vi "testConfigServersAandB.vi"(8 "error in (no error)":errorcluster) -> (0 "error out":errorcluster)   [LabVIEW 2018]
doc: "Test the configServer.vi for TCP/IP servers A and B."
uses:
  src/TcpServer/TcpServer.lvclass
  src/TcpServerTel/typedef/enqueueOptionsTypeDef.ctl
  src/TcpServer/configServerTypeDef.ctl
  src/TcpServer/TcpServer.lvclass/TcpServer.ctl
  src/TcpServerBase/TcpServerBase.lvclass/TcpServerBase.ctl
  src/TcpServerTel/TcpServerTel.lvclass/TcpServerTel.ctl
  src/TcpServerCmd/TcpServerCmd.lvclass
  home/pcortes/Documents/github/ts_labview_tcp_json/src/TcpServerBase/TcpServerBase.lvclass
  src/TcpServerTel/TcpServerTel.lvclass
  <vilib>/addons/_JKI Toolkits/Caraya/classes/Assert/Assert Not Equal Value_Variant.vi
  <vilib>/addons/_JKI Toolkits/Caraya/classes/Assert/Assert Equal Value_Variant.vi
  <vilib>/addons/_JKI Toolkits/Caraya/classes/Test/Test.lvclass
  <vilib>/addons/_JKI Toolkits/Caraya/classes/Assert/Assert.lvclass
  src/TcpServerBase/TcpServerBase.lvclass
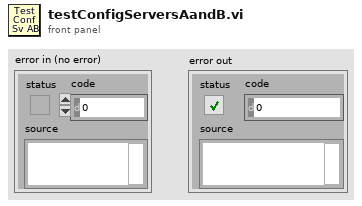
[diagram p1: front panel]
types:
  T1 = typedef "TcpServerTel.lvclass/enqueueOptionsTypeDef.ctl" = enum16{"lossy enqueue", "normal enqueue"}
  T2 = typedef "TcpServer.lvclass/configServerTypeDef.ctl" = cluster{"cmdServerPort":u16, "telServerPort":u16, "timeoutServerInMs":i32, "serverBytesToRead":i32, "maxSizeQueueTcpClientFromDds":i32, "EnqueueOptions":T1, "timeoutQueueTcpClientFromDds (ms)":i32, "maxSizeQueueTcpClient":i32, "timeoutInMs":i32}
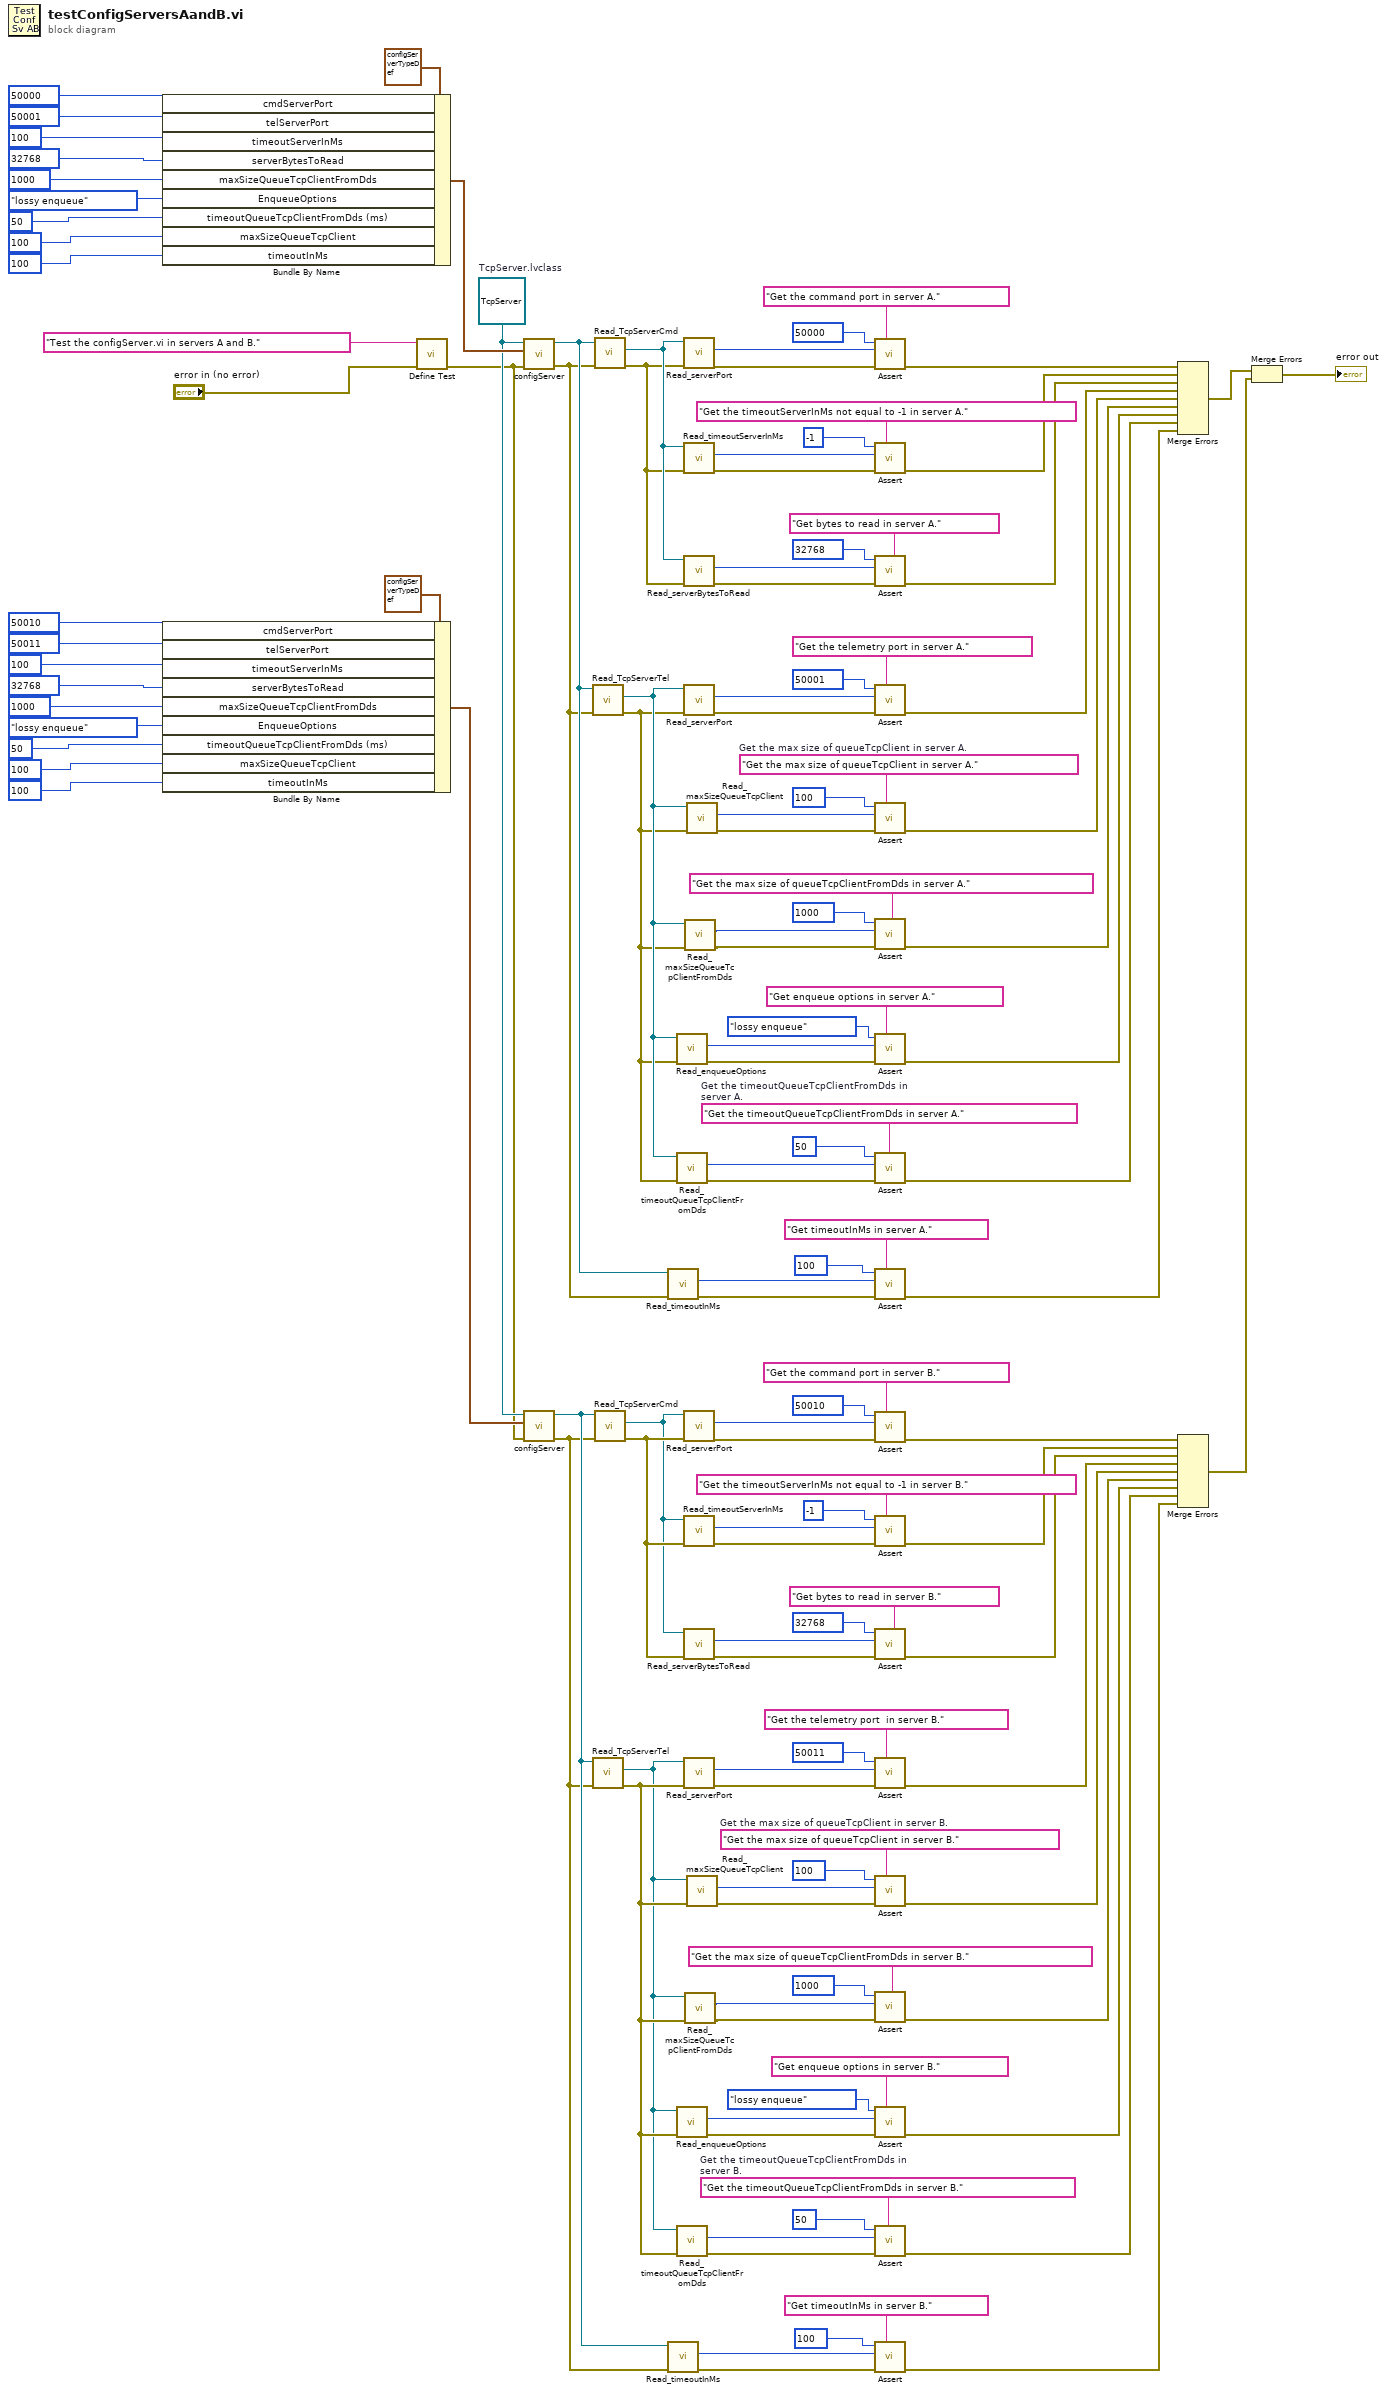
[diagram p0: block diagram]
diagram:
  w34 = "Get the max size of queueTcpClient in server B."  # Get the max size of queueTcpClient in server B.
  w31 = "Get the timeoutQueueTcpClientFromDds in server B."  # Get the timeoutQueueTcpClientFromDds in server B.
  w104 = "Get the max size of queueTcpClient in server A."  # Get the max size of queueTcpClient in server A.
  w107 = "Get the timeoutQueueTcpClientFromDds in server A."  # Get the timeoutQueueTcpClientFromDds in server A.
  w58 = refnum<class "TcpServer.lvclass"> refnum  # TcpServer.lvclass
  n1 = Bundle By Name(cluster=T2 {"cmdServerPort"=8888, "telServerPort"=8889, "timeoutServerInMs"=100, "serverBytesToRead"=32768, "maxSizeQueueTcpClientFromDds"=1000, "EnqueueOptions"=enum."lossy enqueue", "timeoutQueueTcpClientFromDds (ms)"=50, "maxSizeQueueTcpClient"=1000, "timeoutInMs"=100} ("ServerConfiguration"), "cmdServerPort"=u16 50000, "telServerPort"=u16 50001, "timeoutServerInMs"=100 ("serverTimeout (ms)"), "serverBytesToRead"=32768, "maxSizeQueueTcpClientFromDds"=1000 ("telQueueServerMaxSize"), "EnqueueOptions"=enqueueOptionsTypeDef."lossy enqueue", "timeoutQueueTcpClientFromDds (ms)"=50 ("telQueueServerTimeout"), "maxSizeQueueTcpClient"=100 ("tcpClientQueueMaxSize"), "timeoutInMs"=100 ("timeoutStatusNotifier")) -> (w69:T2)
  n2 = Bundle By Name(cluster=T2 {"cmdServerPort"=8888, "telServerPort"=8889, "timeoutServerInMs"=100, "serverBytesToRead"=32768, "maxSizeQueueTcpClientFromDds"=1000, "EnqueueOptions"=enum."lossy enqueue", "timeoutQueueTcpClientFromDds (ms)"=50, "maxSizeQueueTcpClient"=1000, "timeoutInMs"=100} ("ServerConfiguration"), "cmdServerPort"=u16 50010, "telServerPort"=u16 50011, "timeoutServerInMs"=100 ("serverTimeout (ms)"), "serverBytesToRead"=32768, "maxSizeQueueTcpClientFromDds"=1000 ("telQueueServerMaxSize"), "EnqueueOptions"=enqueueOptionsTypeDef."lossy enqueue", "timeoutQueueTcpClientFromDds (ms)"=50 ("telQueueServerTimeout"), "maxSizeQueueTcpClient"=100 ("tcpClientQueueMaxSize"), "timeoutInMs"=100 ("timeoutStatusNotifier")) -> (w8:T2)
  n3 = call <vilib>:"Define Test.vi"("error in (no error)"="error in (no error)", "Label (VI Title)"="Test the configServer.vi in servers A and B.") -> ("error out"=w1:errorcluster)  [unwired: 9 in]
  n4 = call "configServer.vi"("error in (no error)"=w1, "ServerConfiguration"=w69, "tcpServer in"=w58) -> ("error out"=w79:errorcluster, "tcpServer out"=w80:refnum<class "TcpServer.lvclass">)  [unwired: 7 in]
  n5 = call "configServer.vi"("error in (no error)"=w1, "ServerConfiguration"=w8, "tcpServer in"=w58) -> ("error out"=w2:errorcluster, "tcpServer out"=w3:refnum<class "TcpServer.lvclass">)  [unwired: 7 in]
  n6 = call "Read_TcpServerTel.vi"("error in (no error)"=w79, "TcpServer in"=w80) -> ("error out"=w71:errorcluster, "TcpServerTel.lvclass"=w72:refnum<class "TcpServerTel.lvclass">)  [unwired: 7 in, 1 out]
  n7 = call "Read_TcpServerTel.vi"("error in (no error)"=w2, "TcpServer in"=w3) -> ("error out"=w56:errorcluster, "TcpServerTel.lvclass"=w55:refnum<class "TcpServerTel.lvclass">)  [unwired: 7 in, 1 out]
  n8 = call "Read_TcpServerCmd.vi"("error in (no error)"=w79, "TcpServer in"=w80) -> ("error out"=w74:errorcluster, "TcpServerCmd.lvclass"=w75:refnum<class "TcpServerCmd.lvclass">)  [unwired: 7 in, 1 out]
  n9 = call "Read_TcpServerCmd.vi"("error in (no error)"=w2, "TcpServer in"=w3) -> ("error out"=w53:errorcluster, "TcpServerCmd.lvclass"=w52:refnum<class "TcpServerCmd.lvclass">)  [unwired: 7 in, 1 out]
  n10 = call "Read_timeoutInMs.vi"("error in (no error)"=w79, "TcpServer in"=w80) -> ("error out"=w78:errorcluster, "timeoutInMs"=w77:i32)  [unwired: 7 in, 1 out]
  n11 = call "Read_timeoutInMs.vi"("error in (no error)"=w2, "TcpServer in"=w3) -> ("error out"=w49:errorcluster, "timeoutInMs"=w50:i32)  [unwired: 7 in, 1 out]
  n12 = call "Read_enqueueOptions.vi"("error in (no error)"=w71, "TcpServerTel in"=w72) -> ("error out"=w99:errorcluster, "EnqueueOptions"=w98:T1)  [unwired: 7 in, 1 out]
  n13 = call "Read_timeoutQueueTcpClientFromDds.vi"("error in (no error)"=w71, "TcpServerTel in"=w72) -> ("error out"=w97:errorcluster, "timeoutQueueTcpClientFromDds"=w96:i32)  [unwired: 7 in, 1 out]
  n14 = call "Read_enqueueOptions.vi"("error in (no error)"=w56, "TcpServerTel in"=w55) -> ("error out"=w39:errorcluster, "EnqueueOptions"=w40:T1)  [unwired: 7 in, 1 out]
  n15 = call "Read_timeoutQueueTcpClientFromDds.vi"("error in (no error)"=w56, "TcpServerTel in"=w55) -> ("error out"=w41:errorcluster, "timeoutQueueTcpClientFromDds"=w42:i32)  [unwired: 7 in, 1 out]
  n16 = call "Read_serverPort.vi"("error in (no error)"=w74, "TcpServerBase in"=w75) -> ("error out"=w127:errorcluster, "serverPort"=w126:u16)  [unwired: 7 in, 1 out]
  n17 = call "Read_timeoutServerInMs.vi"("error in (no error)"=w74, "TcpServerBase in"=w75) -> ("error out"=w122:errorcluster, "timeoutServerInMs"=w123:i32)  [unwired: 7 in, 1 out]
  n18 = call "Read_serverBytesToRead.vi"("error in (no error)"=w74, "TcpServerBase in"=w75) -> ("error out"=w117:errorcluster, "serverBytesToRead"=w116:i32)  [unwired: 7 in, 1 out]
  n19 = call "Read_serverPort.vi"("error in (no error)"=w71, "TcpServerBase in"=w72) -> ("error out"=w112:errorcluster, "serverPort"=w111:u16)  [unwired: 7 in, 1 out]
  n20 = call "Read_serverPort.vi"("error in (no error)"=w53, "TcpServerBase in"=w52) -> ("error out"=w11:errorcluster, "serverPort"=w12:u16)  [unwired: 7 in, 1 out]
  n21 = call "Read_timeoutServerInMs.vi"("error in (no error)"=w53, "TcpServerBase in"=w52) -> ("error out"=w16:errorcluster, "timeoutServerInMs"=w15:i32)  [unwired: 7 in, 1 out]
  n22 = call "Read_serverBytesToRead.vi"("error in (no error)"=w53, "TcpServerBase in"=w52) -> ("error out"=w21:errorcluster, "serverBytesToRead"=w22:i32)  [unwired: 7 in, 1 out]
  n23 = call "Read_serverPort.vi"("error in (no error)"=w56, "TcpServerBase in"=w55) -> ("error out"=w26:errorcluster, "serverPort"=w27:u16)  [unwired: 7 in, 1 out]
  n24 = call "Read_maxSizeQueueTcpClientFromDds.vi"("error in (no error)"=w71, "TcpServerTel in"=w72) -> ("error out"=w101:errorcluster, "maxSizeQueueTcpClientFromDds"=w100:i32)  [unwired: 7 in, 1 out]
  n25 = call "Read_maxSizeQueueTcpClientFromDds.vi"("error in (no error)"=w56, "TcpServerTel in"=w55) -> ("error out"=w37:errorcluster, "maxSizeQueueTcpClientFromDds"=w38:i32)  [unwired: 7 in, 1 out]
  n26 = call "Read_maxSizeQueueTcpClient.vi"("error in (no error)"=w71, "TcpServerBase in"=w72) -> ("error out"=w103:errorcluster, "maxSizeQueueTcpClient"=w102:i32)  [unwired: 7 in, 1 out]
  n27 = call "Read_maxSizeQueueTcpClient.vi"("error in (no error)"=w56, "TcpServerBase in"=w55) -> ("error out"=w35:errorcluster, "maxSizeQueueTcpClient"=w36:i32)  [unwired: 7 in, 1 out]
  n28 = call-poly <vilib>:"Assert.vi"("Label"="Get the command port in server A.", "error in (no error)"=w127, "Y"=w126, "X"=50000) -> ("error out"=w121:errorcluster)  [unwired: 7 in]
  n29 = call-poly <vilib>:"Assert.vi"("Label"="Get the timeoutServerInMs not equal to -1 in server A.", "error in (no error)"=w122, "Y"=w123, "X"=-1) -> ("error out"=w120:errorcluster)  [unwired: 7 in]
  n30 = call-poly <vilib>:"Assert.vi"("Label"="Get bytes to read in server A.", "error in (no error)"=w117, "Y"=w116, "X"=32768) -> ("error out"=w115:errorcluster)  [unwired: 7 in]
  n31 = call-poly <vilib>:"Assert.vi"("Label"="Get the telemetry port in server A.", "error in (no error)"=w112, "Y"=w111, "X"=50001) -> ("error out"=w73:errorcluster)  [unwired: 7 in]
  n32 = call-poly <vilib>:"Assert.vi"("Label"=w104, "error in (no error)"=w103, "Y"=w102, "X"=100) -> ("error out"=w95:errorcluster)  [unwired: 7 in]
  n33 = call-poly <vilib>:"Assert.vi"("Label"="Get the max size of queueTcpClientFromDds in server A.", "error in (no error)"=w101, "Y"=w100, "X"=1000) -> ("error out"=w94:errorcluster)  [unwired: 7 in]
  n34 = call-poly <vilib>:"Assert.vi"("Label"="Get enqueue options in server A.", "error in (no error)"=w99, "Y"=w98, "X"=enqueueOptionsTypeDef."lossy enqueue" ("EnqueueOptions")) -> ("error out"=w93:errorcluster)  [unwired: 7 in]
  n35 = call-poly <vilib>:"Assert.vi"("Label"=w107, "error in (no error)"=w97, "Y"=w96, "X"=50) -> ("error out"=w92:errorcluster)  [unwired: 7 in]
  n36 = call-poly <vilib>:"Assert.vi"("Label"="Get timeoutInMs in server A.", "error in (no error)"=w78, "Y"=w77, "X"=100) -> ("error out"=w70:errorcluster)  [unwired: 7 in]
  n37 = call-poly <vilib>:"Assert.vi"("Label"="Get the command port in server B.", "error in (no error)"=w11, "Y"=w12, "X"=50010) -> ("error out"=w17:errorcluster)  [unwired: 7 in]
  n38 = call-poly <vilib>:"Assert.vi"("Label"="Get the timeoutServerInMs not equal to -1 in server B.", "error in (no error)"=w16, "Y"=w15, "X"=-1) -> ("error out"=w18:errorcluster)  [unwired: 7 in]
  n39 = call-poly <vilib>:"Assert.vi"("Label"="Get bytes to read in server B.", "error in (no error)"=w21, "Y"=w22, "X"=32768) -> ("error out"=w23:errorcluster)  [unwired: 7 in]
  n40 = call-poly <vilib>:"Assert.vi"("Label"="Get the telemetry port  in server B.", "error in (no error)"=w26, "Y"=w27, "X"=50011) -> ("error out"=w54:errorcluster)  [unwired: 7 in]
  n41 = call-poly <vilib>:"Assert.vi"("Label"=w34, "error in (no error)"=w35, "Y"=w36, "X"=100) -> ("error out"=w43:errorcluster)  [unwired: 7 in]
  n42 = call-poly <vilib>:"Assert.vi"("Label"="Get the max size of queueTcpClientFromDds in server B.", "error in (no error)"=w37, "Y"=w38, "X"=1000) -> ("error out"=w44:errorcluster)  [unwired: 7 in]
  n43 = call-poly <vilib>:"Assert.vi"("Label"="Get enqueue options in server B.", "error in (no error)"=w39, "Y"=w40, "X"=enqueueOptionsTypeDef."lossy enqueue" ("EnqueueOptions")) -> ("error out"=w45:errorcluster)  [unwired: 7 in]
  n44 = call-poly <vilib>:"Assert.vi"("Label"=w31, "error in (no error)"=w41, "Y"=w42, "X"=50) -> ("error out"=w46:errorcluster)  [unwired: 7 in]
  n45 = call-poly <vilib>:"Assert.vi"("Label"="Get timeoutInMs in server B.", "error in (no error)"=w49, "Y"=w50, "X"=100) -> ("error out"=w57:errorcluster)  [unwired: 7 in]
  n46 = Merge Errors(w121, w120, w115, w73, w95, w94, w93, w92, w70) -> (w6:errorcluster)
  n47 = Merge Errors(w17, w18, w23, w54, w43, w44, w45, w46, w57) -> (w5:errorcluster)
  n48 = Merge Errors(w6, w5) -> (→"error out":errorcluster)
